vi "2016110576강재원_2번Project.vi"() -> ()   [LabVIEW 2017]
uses:
  <vilib>/DAQmx/miscellaneous.llb/DAQmx Fill In Error Info.vi
  <vilib>/DAQmx/create/channels.llb/DAQmx Create Channel (CO-Pulse Generation-Frequency).vi
  <vilib>/DAQmx/create/channels.llb/DAQmx Create Channel (AI-Voltage-Basic).vi
  <vilib>/DAQmx/configure/timing.llb/DAQmx Timing (Implicit).vi
  <vilib>/DAQmx/create/channels.llb/DAQmx Create Channel (DO-Digital Output).vi
  <vilib>/DAQmx/write.llb/DAQmx Write (Counter Frequency 1Chan 1Samp).vi
  <vilib>/DAQmx/read.llb/DAQmx Read (Analog DBL 1Chan 1Samp).vi
  <vilib>/DAQmx/write.llb/DAQmx Write (Digital Bool 1Line 1Point).vi
panel:
  out "물고기의 건강":u8(slide) caption="물고기의 스트레스" scale=0.0..100.0
  out "물고기의 스트레스":u8(slide) scale=0.0..5.0
  out "제어LED밝기(0.01~0.99)":dbl
  in  "밝기제어\nON/OFF":bool
  in  "포텐쇼led,0번핀":tag
  in  "PWMled, 카운터":tag
  in  "정지":bool
  in  "조도센서, 아날로그0번":tag
  out "수조의 밝기":dbl(graph)
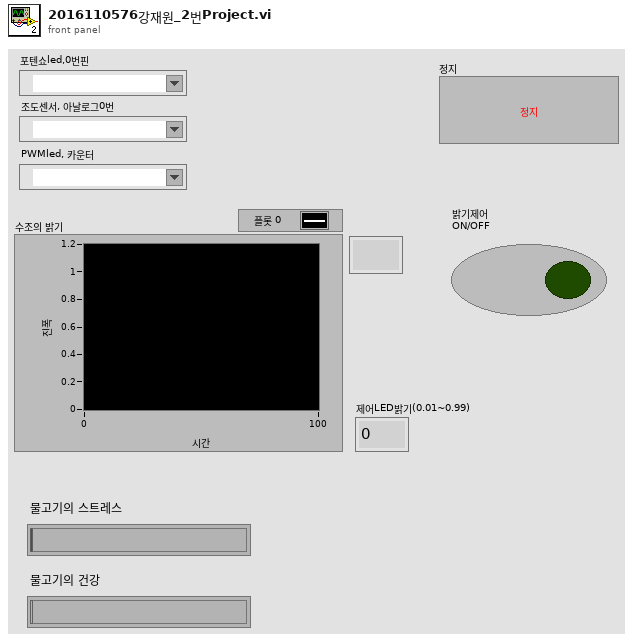
[diagram p1: front panel]
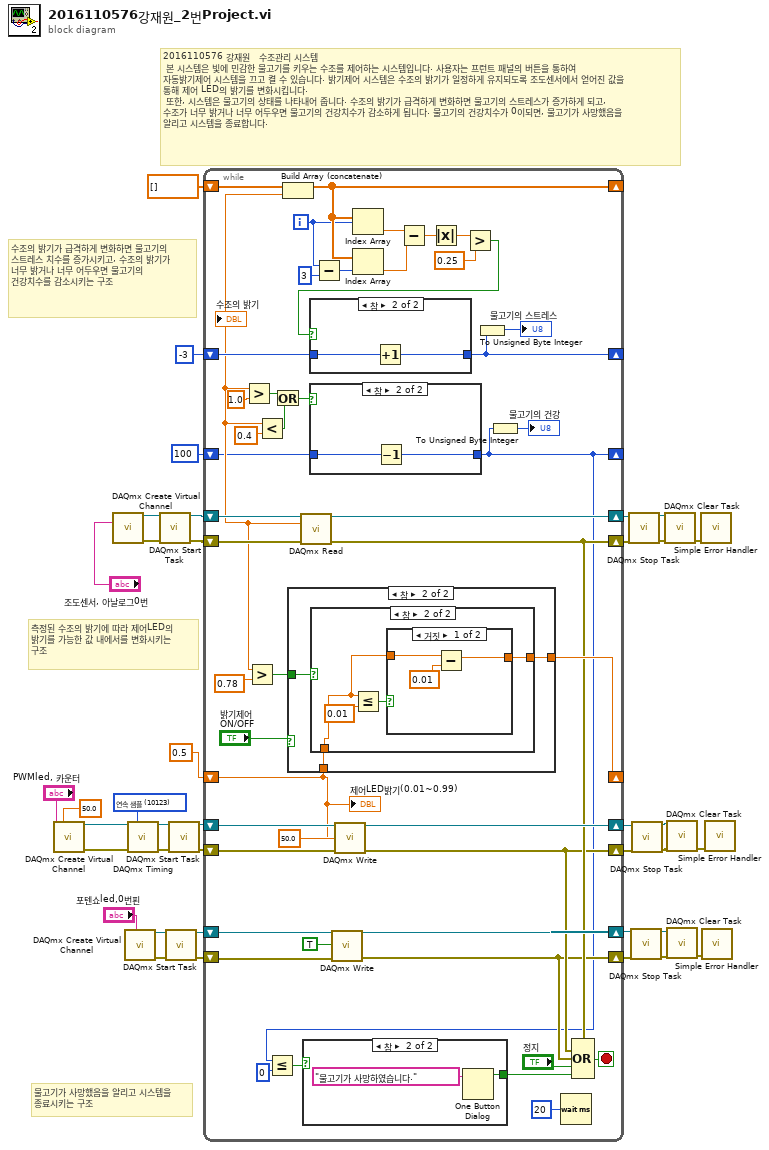
[diagram p0: block diagram]
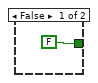
[diagram p2: hidden frame]
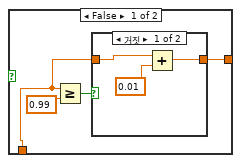
[diagram p6: hidden frame]
diagram:
  w20 = 10123 items=["유한 샘플"=10178, "연속 샘플"=10123, "하드웨어 타이밍에 의한 단일 포인트"=12522] ("sample mode")
  # "수조의 밝기가 급격하게 변화하면 물고기의 스트레스 치수를 증가시키고, 수조의 밝기가 너무 밝거나 너무 어두우면 물고기의 건강치수를 감소시키는 구조"
  # "측정된 수조의 밝기에 따라 제어LED의 밝기를 가능한 값 내에서를 변화시키는 구조"
  # "물고기가 사망했음을 알리고 시스템을 종료시키는 구조"
  # "2016110576 강재원   수조관리 시스템\n 본 시스템은 빛에 민감한 물고기를 키우는 수조를 제어하는 시스템입니다. 사용자는 프런트 패널의 버튼을 통하여 자동밝기제어 시스템을 끄고 켤 수 있습니다. 밝기제어 시스템은 수조의 밝기가 일정하게 유지되도록 조도센서에서 얻어진 값을 통해 제어 LED의 밝기를 변화시킵니다. \n 또한, 시스템은 물고기의 상태를 나타내어 줍니다. 수조의 밝기가 급격하게 변화하면 물고기의 스트레스가 증가하게 되고, 수조가 너무 밝거나 너무 어두우면 물고기의 건강치수가 감소하게 됩니다. 물고기의 건강치수가 0이되면, 물고기가 사망했음을 알리고 시스템을 종료합니다."
  n1 = call-poly <vilib>:"DAQmx Create Virtual Channel.vi"("frequency"=50.0, "counter"="PWMled, 카운터") -> ("task out"=w29:refnum<k21>, "error out"=w28:errorcluster)  [unwired: 12 in]
  n2 = call-poly <vilib>:"DAQmx Create Virtual Channel.vi"("physical channels"="조도센서, 아날로그0번") -> ("task out"=w31:refnum<k21>, "error out"=w30:errorcluster)  [unwired: 13 in]
  n3 = call-poly <vilib>:"DAQmx Create Virtual Channel.vi"("lines"="포텐쇼led,0번핀") -> ("task out"=w7:refnum<k21>, "error out"=w8:errorcluster)  [unwired: 13 in]
  n4 = call-poly <vilib>:"DAQmx Timing.vi"("task/channels in"=w29, "sample mode"=w20, "error in"=w28) -> ("task out"=w26:refnum<k21>, "error out"=w27:errorcluster)  [unwired: 11 in]
  n5 = call <vilib>:"DAQmx Start Task.vi"("task/channels in"=w31, "error in"=w30) -> ("task out"=w32:refnum<k21>, "error out"=w33:errorcluster)  [unwired: 12 in]
  n6 = call <vilib>:"DAQmx Start Task.vi"("task/channels in"=w7, "error in"=w8) -> ("task out"=w9:refnum<k21>, "error out"=w10:errorcluster)  [unwired: 12 in]
  n7 = call <vilib>:"DAQmx Start Task.vi"("task/channels in"=w26, "error in"=w27) -> ("task out"=w25:refnum<k21>, "error out"=w24:errorcluster)  [unwired: 12 in]
  n8 = while {
    shift-right: [w84] -> w35
    shift-left: w32 -> [w85]
    shift-right: [w46] -> w36
    shift-left: w33 -> [w86]
    shift-right: [w81] -> w23
    shift-left: w25 -> [w83]
    shift-right: [w45] -> w22
    shift-left: w24 -> [w82]
    shift-right: [w79] -> w12
    shift-left: w9 -> [w77]
    shift-right: [w43] -> w11
    shift-left: w10 -> [w78]
    shift-right: [w72] -> _
    shift-left: 0.5 -> [w73]
    shift-right: [w69] -> _
    shift-left: dbl[] [] -> [w70]
    shift-right: [w59] -> _
    shift-left: -3 -> [w61]
    shift-right: [w41] -> _
    shift-left: 100 -> [w51]
    i -> [w58]
    stop <- w47 stop-if-true
    n9 = call-poly <vilib>:"DAQmx Read.vi"("task/channels in"=w85, "error in"=w86) -> ("task out"=w84:refnum<k21>, "data"=w53:dbl, "error out"=w46:errorcluster)  [unwired: 11 in]
    "수조의 밝기" <- w53
    n10 = Greater?(x=w53, y=1.0) -> (0:w55:bool)
    n11 = Greater?(x=w53, y=0.78) -> (0:w74:bool)
    n12 = Less?(x=w53, y=0.4) -> (x < y?=w54:bool)
    n13 = Or(x=w55, y=w54) -> (x .or. y?=w52:bool)
    n14 = Build Array (concatenate)(w70, w53) -> (w69:dbl[])
    n15 = case shown="참" "밝기제어\nON/OFF" {
      tunnel: w74 -> [_ w99]
      tunnel: w73 -> [w96 w98]
      tunnel: [w96 w97] -> w72
      frame False {
      }
      frame True {
        n16 = case shown="참" w99 {
          tunnel: w98 -> [w100 w109]
          tunnel: [w102 w108] -> w97
          frame False {
            n17 = Greater Or Equal?(x=w100, y=0.99) -> (x >= y?=w101:bool)
            n18 = case shown="거짓" w101 {
              tunnel: [w105 w107] -> w102
              tunnel: w100 -> [w104 w107]
              frame False {
                n19 = Add(x=w104, y=0.01) -> (x+y=w105:dbl)
              }
              frame True {
              }
            }
          }
          frame True {
            n20 = Less Or Equal?(x=w109, y=0.01) -> (x <= y?=w110:bool)
            n21 = case shown="거짓" w110 {
              tunnel: w109 -> [w114 w115]
              tunnel: [w112 w115] -> w108
              frame False {
                n22 = Subtract(x=w114, y=0.01) -> (x-y=w112:dbl)
              }
              frame True {
              }
            }
          }
        }
      }
    }
    n23 = case shown="참" w52 {
      tunnel: w51 -> [w90 w92]
      tunnel: [w90 w91] -> w41
      frame False {
      }
      frame True {
        n24 = Decrement(x=w92) -> (x-1=w91:i32)
      }
    }
    n25 = Less Or Equal?(x=w41, y=0) -> (x <= y?=w39:bool)
    n26 = case shown="참" w39 {
      tunnel: [FALSE w89] -> w42
      frame False {
      }
      frame True {
        n27 = One Button Dialog(message="물고기가 사망하였습니다." ("메시지")) -> (true=w89:bool)  [unwired: 1 in]
      }
    }
    n28 = Subtract(x=w58, y=3) -> (x-y=w68:i32)
    n29 = call-poly <vilib>:"DAQmx Write.vi"("task/channels in"=w77, "data"=TRUE, "error in"=w78) -> ("task out"=w79:refnum<k21>, "error out"=w43:errorcluster)  [unwired: 10 in, 1 out]
    n30 = call-poly <vilib>:"DAQmx Write.vi"("task/channels in"=w83, "frequency"=50.0, "duty cycle"=w73, "error in"=w82) -> ("task out"=w81:refnum<k21>, "error out"=w45:errorcluster)  [unwired: 9 in, 1 out]
    n31 = Index Array(array=w69, index=w58) -> (element=w67:dbl)
    n32 = Index Array(array=w69, index=w68) -> (element=w66:dbl)
    n33 = Subtract(x=w67, y=w66) -> (x-y=w65:dbl)
    n34 = Absolute Value(x=w65) -> (abs(x)=w64:dbl)
    n35 = Greater?(x=w64, y=0.25) -> (0:w62:bool)
    n36 = case shown="참" w62 {
      tunnel: w61 -> [w93 w95]
      tunnel: [w93 w94] -> w59
      frame False {
      }
      frame True {
        n37 = Increment(x=w95) -> (x+1=w94:i32)
      }
    }
    n38 = To Unsigned Byte Integer(number=w59) -> (unsigned 8bit integer=→"물고기의 스트레스":u8)
    n39 = To Unsigned Byte Integer(number=w41) -> (unsigned 8bit integer=→"물고기의 건강":u8)
    n40 = Wait (ms)(milliseconds to wait=u32 20 ("대기 시간 (ms)")) -> ()  [unwired: 1 out]
    n41 = Compound Arithmetic op=OR ("복합 연산")(w46, w45, w43, "정지", w42) -> (w47:bool)
    "제어LED밝기(0.01~0.99)" <- w73
  }
  n42 = call <vilib>:"DAQmx Stop Task.vi"("task/channels in"=w35, "error in"=w36) -> ("task out"=w34:refnum<k21>, "error out"=w37:errorcluster)  [unwired: 12 in]
  n43 = call <vilib>:"DAQmx Stop Task.vi"("task/channels in"=w12, "error in"=w11) -> ("task out"=w14:refnum<k21>, "error out"=w15:errorcluster)  [unwired: 12 in]
  n44 = call <vilib>:"DAQmx Stop Task.vi"("task/channels in"=w23, "error in"=w22) -> ("task out"=w19:refnum<k21>, "error out"=w21:errorcluster)  [unwired: 12 in]
  n45 = call <vilib>:"DAQmx Clear Task.vi"("task in"=w34, "error in"=w37) -> ("error out"=w38:errorcluster)  [unwired: 13 in]
  n46 = call <vilib>:"DAQmx Clear Task.vi"("task in"=w19, "error in"=w21) -> ("error out"=w18:errorcluster)  [unwired: 13 in]
  n47 = call <vilib>:"DAQmx Clear Task.vi"("task in"=w14, "error in"=w15) -> ("error out"=w13:errorcluster)  [unwired: 13 in]
  n48 = call <vilib>:"Simple Error Handler.vi"("error in (no error)"=w38) -> ()  [unwired: 4 in, 5 out]
  n49 = call <vilib>:"Simple Error Handler.vi"("error in (no error)"=w13) -> ()  [unwired: 4 in, 5 out]
  n50 = call <vilib>:"Simple Error Handler.vi"("error in (no error)"=w18) -> ()  [unwired: 4 in, 5 out]
